vi "ingest.mcap_set_ignore_invalid_topics.vi"(8 "error in":errorcluster, 11 "McapIngestStaging in":refnum<class "McapIngestStaging.lvclass">) -> (0 "error out":errorcluster, 3 "McapIngestStaging out":refnum<class "McapIngestStaging.lvclass">)   [LabVIEW 2020, in "McapIngestStaging.lvclass"]
doc: "Chooses whether invalid MCAP topics are skipped instead of failing the whole ingest."
uses:
  McapIngestStaging.lvclass
  McapIngestStaging.lvclass/McapIngestStaging.ctl
  client.lvlib
panel:
  in  "ignore":bool
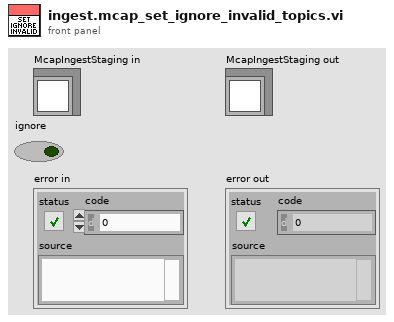
[diagram p1: front panel]
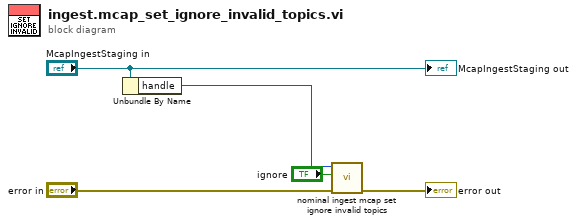
[diagram p0: block diagram]
diagram:
  n1 = Unbundle By Name("McapIngestStaging in") -> ("handle"=w3:i32)
  n2 = call "nominal ingest mcap set ignore invalid topics.vi"("error in (no error)"="error in", "ignore"="ignore", "staging"=w3) -> ("error out"=→"error out":errorcluster)  [unwired: 7 in, 1 out]
  "McapIngestStaging out" <- "McapIngestStaging in"
